vi "Read_from_Flash.vi"() -> (0 "correction":dbl[](array[numeric]))   [LabVIEW 2022 SP3]
uses:
  adcDLL_0001.dll
panel:
  out "Waveform Graph 2":dbl[](graph)
  in  "address 2":u32
  in  "DevDet":i32=1
  in  "address":u32=1
  out "initialized array":u8[](array[numeric])
  out "InputData1":u8[](array[numeric])
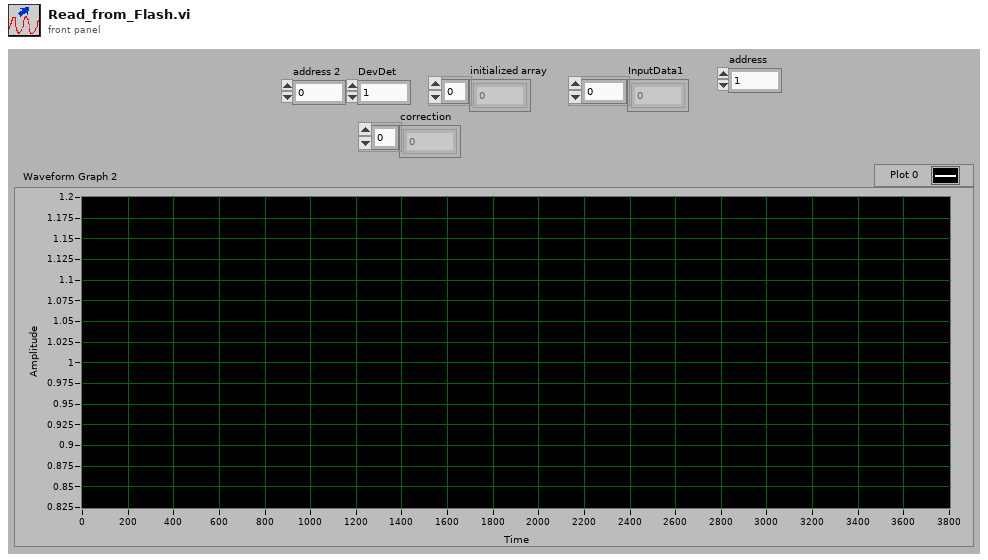
[diagram p1: front panel]
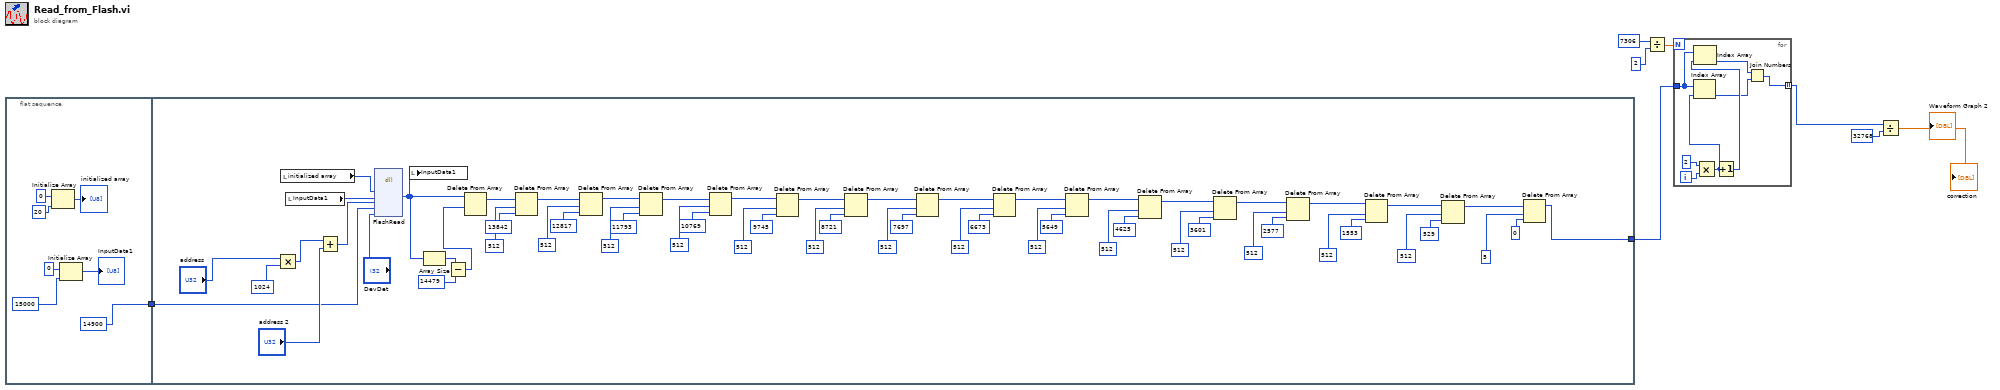
[diagram p0: block diagram]
diagram:
  n1 = flat-sequence {
    tunnel: [14900 ("dimension size")] -> w8
    tunnel: w8 -> [w66]
    tunnel: [w16] -> w7
    frame #0 {
      n2 = Initialize Array(u8 0 ("element"), 20 ("dimension size")) -> (→"initialized array":u8[])
      n3 = Initialize Array(u8 0 ("element"), 15000 ("dimension size")) -> (→"InputData1":u8[])
    }
    frame #1 {
      n4 = Multiply(x="address", y=u32 1024) -> (x*y=w69:u32)
      n5 = local read "initialized array"() -> (w74:u8[])
      n6 = local read "InputData1"() -> (w73:u8[])
      n7 = Add(x=w69, y="address 2") -> (x+y=w71:u32)
      n8 = dll-call lib="D:/LabVIEWSuite_64_OS/Spectrometers/ASEQ LR1/adcDLL_0001.dll" fn="FlashRead"("OutputReport1"=w74, "InputData1"=w73, "address"=w71, "length"=w66, "DevDet"="DevDet") -> ("InputData1"=w65:u8[])  [unwired: 8 in, 2 out]
      n9 = local write "InputData1"(w65) -> ()
      n10 = Array Size(array=w65) -> (size(s)=w64:i32)
      n11 = Subtract(x=w64, y=14479) -> (x-y=w62:i32)
      n12 = Delete From Array(array=w65, length=w62) -> (array with subset deleted=w31:u8[])  [unwired: 1 in, 1 out]
      n13 = Delete From Array(array=w31, length=512, index=13842) -> (array with subset deleted=w30:u8[])  [unwired: 1 out]
      n14 = Delete From Array(array=w30, length=512, index=12817) -> (array with subset deleted=w29:u8[])  [unwired: 1 out]
      n15 = Delete From Array(array=w29, length=512, index=11793) -> (array with subset deleted=w28:u8[])  [unwired: 1 out]
      n16 = Delete From Array(array=w28, length=512, index=10769) -> (array with subset deleted=w27:u8[])  [unwired: 1 out]
      n17 = Delete From Array(array=w27, length=512, index=9745) -> (array with subset deleted=w26:u8[])  [unwired: 1 out]
      n18 = Delete From Array(array=w26, length=512, index=8721) -> (array with subset deleted=w25:u8[])  [unwired: 1 out]
      n19 = Delete From Array(array=w25, length=512, index=7697) -> (array with subset deleted=w24:u8[])  [unwired: 1 out]
      n20 = Delete From Array(array=w24, length=512, index=6673) -> (array with subset deleted=w23:u8[])  [unwired: 1 out]
      n21 = Delete From Array(array=w23, length=512, index=5649) -> (array with subset deleted=w22:u8[])  [unwired: 1 out]
      n22 = Delete From Array(array=w22, length=512, index=4625) -> (array with subset deleted=w21:u8[])  [unwired: 1 out]
      n23 = Delete From Array(array=w21, length=512, index=3601) -> (array with subset deleted=w20:u8[])  [unwired: 1 out]
      n24 = Delete From Array(array=w20, length=512, index=2577) -> (array with subset deleted=w19:u8[])  [unwired: 1 out]
      n25 = Delete From Array(array=w19, length=512, index=1553) -> (array with subset deleted=w18:u8[])  [unwired: 1 out]
      n26 = Delete From Array(array=w18, length=512, index=529) -> (array with subset deleted=w17:u8[])  [unwired: 1 out]
      n27 = Delete From Array(array=w17, length=5, index=0) -> (array with subset deleted=w16:u8[])  [unwired: 1 out]
    }
  }
  n28 = Divide(x=7306 ("dimension size"), y=2) -> (x/y=w6:dbl)
  n29 = for {
    N: w6 -> [_]
    tunnel: w7 -> [w79]
    tunnel: [w75] -> w2 mode=indexing
    i -> [w82]
    n30 = Multiply(x=2, y=w82) -> (x*y=w80:i32)
    n31 = Index Array(array=w79, index=w80) -> (element=w77:u8)
    n32 = Increment(x=w80) -> (x+1=w78:i32)
    n33 = Index Array(array=w79, index=w78) -> (element=w76:u8)
    n34 = Join Numbers(hi=w76, lo=w77) -> ((hi.lo)=w75:u16)
  }
  n35 = Divide(x=w2, y=u16 32768) -> (x/y=→"Waveform Graph 2" →"correction":dbl[])
